vi "RunMacro.vi"(5 "abs. path":bool=TRUE, 6 "sequence folder":path, 7 "submacro":bool, 8 "error in (no error)":errorcluster, 9 "platform":u16(ring) items=["Mac", "PC"], 10 "Message_command":T1={"No. of command"=0, "Parameters"=[], "Address"="", "Boolean"=TRUE, "No. of line"=0, "Initial Time"=timestamp(0 s since 1904-01-01), "Current Time"=timestamp(0 s since 1904-01-01), "Sequence status"="", "Sequence"=refnum, "Temp_Check"=0, "Sequence_History"="", "Subsequence"=[]}, 11 "queue":refnum<queue>) -> (0 "error out":errorcluster, 2 "macro name":string, 3 "queue out":refnum<queue>)   [LabVIEW 2025]
uses:
  <vilib>/Utility/file.llb/Read Delimited Spreadsheet (string).vi
panel:
  out "No. of line":i32
  in  "resume":enum16{"none", "paused", "skipped"}(ring)
  in  "allow recursive":bool
  in  "restart line":i32
  in  "Subseq":i32[](listbox)=[4] caption="subseq"
  out "Path":path=path "C:/Users/shared/Sequences/MPMS_LCR_Tsweep.vi.txt"
  # "Shows the current running macro including\nthe submacros line by line."
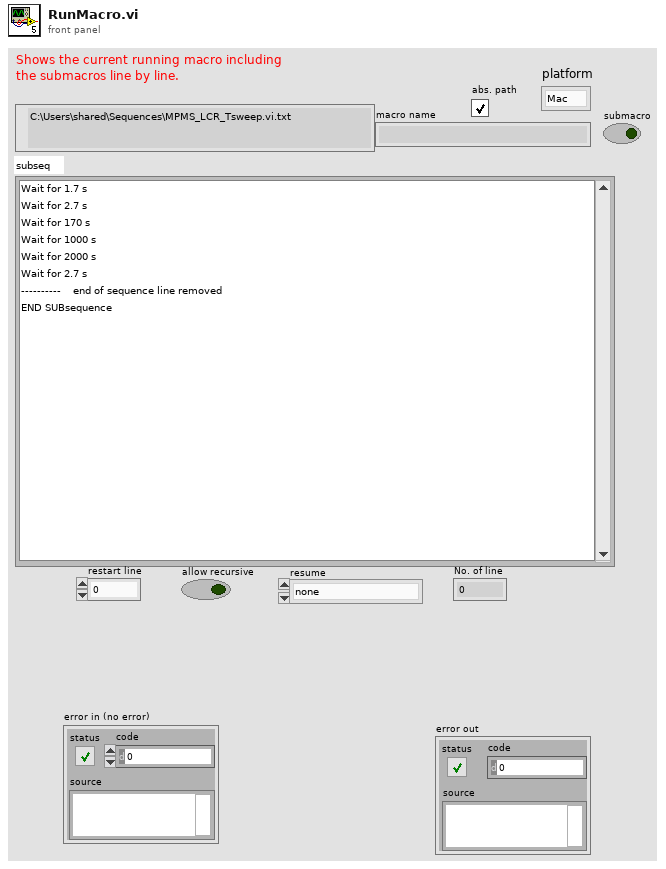
[diagram p1: front panel]
types:
  T1 = cluster{"No. of command":i32, "Parameters":string[], "Address":refnum<visa-resource-name>, "Boolean":bool, "No. of line":i32, "Initial Time":timestamp, "Current Time":timestamp, "Sequence status":string, "Sequence":refnum<vi>, "Temp_Check":i32, "Sequence_History":string, "Subsequence":string[]}
  T2 = typedef "Command_Message.ctl" = cluster{"No. of command":i32, "Parameters":string[], "Address":refnum<visa-resource-name>, "Boolean":bool, "No. of line":i32, "Initial Time":timestamp, "Current Time":timestamp, "Status":string, "Sequence Ref.":refnum<vi>, "Temp check":i32, "Sequence_History":string, "Subsequence":string[]}
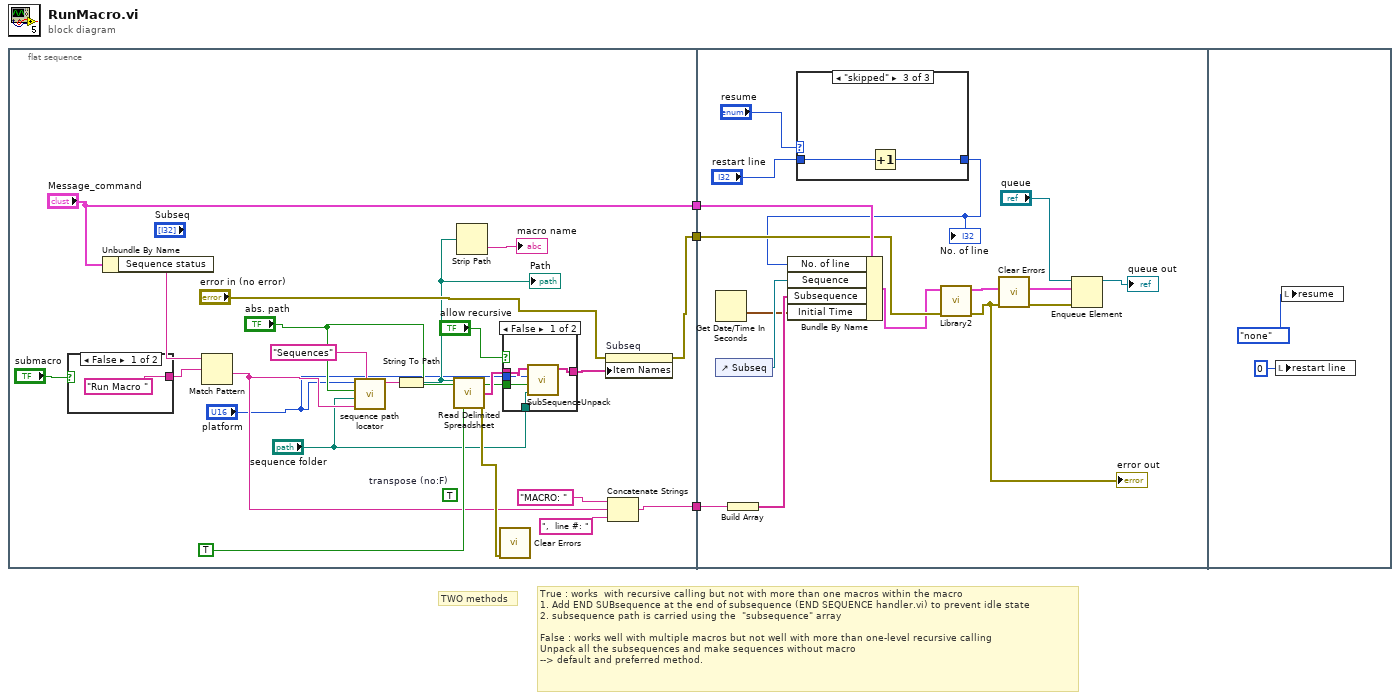
[diagram p0: block diagram]
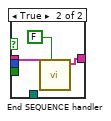
[diagram p2: hidden frame]
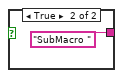
[diagram p3: hidden frame]
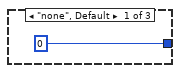
[diagram p4: hidden frame]
diagram:
  # "TWO methods"
  # "True : works  with recursive calling but not with more than one macros within the macro\n1. Add END SUBsequence at the end of subsequence (END SEQUENCE handler.vi) to prevent idle state\n2. subsequence path is carried using the  \"subsequence\" array\n\nFalse : works well with multiple macros but not well with more than one-level recursive calling\nUnpack all the subsequences and make sequences without macro\n--> default and preferred method."
  n1 = flat-sequence {
    tunnel: ["Message_command"] -> w3
    tunnel: [w22] -> w2
    tunnel: [w17] -> w1
    tunnel: w3 -> [w46]
    tunnel: w2 -> [w45]
    tunnel: w1 -> [w43]
    frame #0 {
      (unwired) TRUE  # transpose (no:F)
      n2 = case shown="False" "submacro" {
        tunnel: ["Run Macro " ("regular expression") "SubMacro " ("regular expression")] -> w23
        frame False {
        }
        frame True {
        }
      }
      n3 = Unbundle By Name("Message_command") -> ("Sequence status"=w19:string)
      n4 = Match Pattern(string=w19, regular expression=w23) -> (after substring=w10:string)  [unwired: 1 in, 3 out]
      n5 = call "sequence path locator.vi"("Sequence folder name"="Sequences", "sequence path"=w10, "Sequences folder path"="sequence folder", "Use absolute sequence path"="abs. path", "platform"="platform") -> ("modified path"=w8:string)  [unwired: 6 in]
      n6 = String To Path(string=w8) -> (path=w11:path)
      "Path" <- w11
      n7 = call-poly <vilib>:"Read Delimited Spreadsheet.vi"("file path (dialog if empty)"=w11, "transpose? (F)"=TRUE) -> ("first row"=w13:string[], "error out"=w12:errorcluster)  [unwired: 8 in, 4 out]
      n8 = Strip Path(path=w11) -> (name=→"macro name":string)  [unwired: 1 out]
      n9 = call <vilib>:"Clear Errors.vi"("error in (no error)"=w12) -> ()  [unwired: 5 in, 2 out]
      n10 = case shown="False" "allow recursive" {
        tunnel: w13 -> [w30 w33]
        tunnel: [w29 w32] -> w21
        tunnel: "abs. path" -> [w28 _]
        tunnel: "sequence folder" -> [w27 _]
        tunnel: "platform" -> [w26 _]
        frame False {
          n11 = call "SubSequenceUnpack.vi"("Sequences folder path"=w27, "Use absolute sequence path"=w28, "platform"=w26, "input sequences"=w30) -> ("output sequences"=w29:string[])  [unwired: 7 in]
        }
        frame True {
          n12 = call "End SEQUENCE handler.vi"("main seq?"=FALSE, "input sequences"=w33) -> ("output sequences"=w32:string[])  [unwired: 9 in]
        }
      }
      n13 = property on="Subseq" class="LstBox (strict)"(error in="error in (no error)", "Item Names"=w21) -> (error out=w22:errorcluster)  [unwired: 1 in, 1 out]
      n14 = Concatenate Strings("MACRO: " ("string"), w10, ",  line #: " ("string")) -> (w17:string)
    }
    frame #1 {
      n15 = Get Date/Time In Seconds() -> (seconds since 1Jan1904=w36:timestamp)
      n16 = control-ref of="Subseq"() -> (w47:refnum<vi>)
      n17 = Build Array(w43) -> (w44:string[])
      n18 = case shown="\"skipped\"" "resume" {
        tunnel: [0 ("No. of line") w52 w53] -> w40
        tunnel: "restart line" -> [_ w52 w54]
        frame "none", Default {
        }
        frame "paused" {
        }
        frame "skipped" {
          n19 = Increment(x=w54) -> (x+1=w53:i32)
        }
      }
      "No. of line" <- w40
      n20 = Bundle By Name(cluster=w46, "No. of line"=w40, "Sequence"=w47, "Subsequence"=w44, "Initial Time"=w36) -> (w37:T1)
      n21 = call "Library2.vi"("Message_command_in"=w37, "error in (no error)"=w45) -> ("Message_command out"=w50:T2, "error out"=w41:errorcluster)  [unwired: 7 in]
      "error out" <- w41
      n22 = call <vilib>:"Clear Errors.vi"("error in (no error)"=w41) -> ("error out"=w42:errorcluster)  [unwired: 5 in, 1 out]
      n23 = Enqueue Element(queue="queue", element=w50, error in (no error)=w42) -> (queue out=→"queue out":refnum<queue>)  [unwired: 1 in, 2 out]
    }
    frame #2 {
      n24 = local write "restart line"(0 ("restart line")) -> ()
      n25 = local write "resume"(enum16{"none", "paused", "skipped"}."none" ("resume")) -> ()
    }
  }
